vi "Convert Channels to Configuration.vi"(8 "error in":errorcluster, 10 "Conversion time":u32, 11 "Channels":T3(array[cluster]) {"RTD type" items=["User Defined"=0, "TCR3750"=2, "TCR3851"=7]}) -> (0 "error out":errorcluster, 3 "_9226 Config Data":T1 {"RTD_Type" items=["User Defined"=0, "TCR3750"=2, "TCR3851"=7]; "Degree Range" items=["Raw Ohms", "Degrees Kelvin", "Degrees Celsius", "Degrees Fahrenheit", "Degrees Rankine"]; "Conversion Time" items=["200 ms", "2.5 ms"]})   [LabVIEW 2019, in "Modules.lvlib" / "9226.lvclass"]
uses:
  9226.lvclass
  Supported RTD Types.ctl
  9226 Configuration.ctl
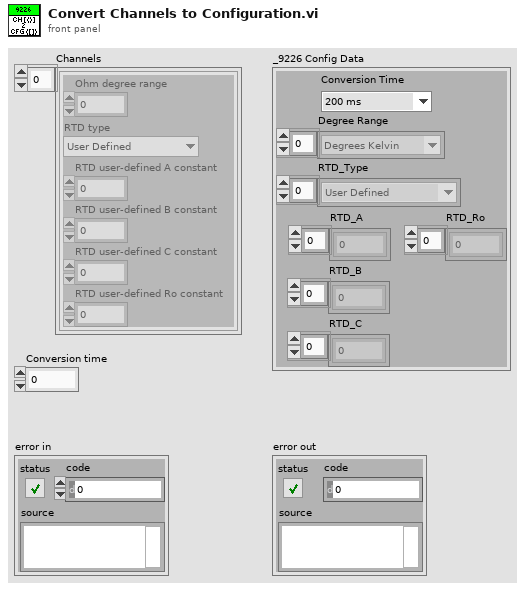
[diagram p1: front panel]
types:
  T1 = typedef "Modules.lvlib/9226.lvclass/9226 Configuration.ctl" = cluster{"Conversion Time":u16, "Degree Range":u32[], "RTD_Type":T2[], "RTD_A":dbl[], "RTD_B":dbl[], "RTD_C":dbl[], "RTD_Ro":dbl[]}
  T2 = typedef "Modules.lvlib/9226.lvclass/Supported RTD Types.ctl" = u32
  T3 = cluster{"Ohm degree range":u32, "RTD type":T2, "RTD user-defined A constant":dbl, "RTD user-defined B constant":dbl, "RTD user-defined C constant":dbl, "RTD user-defined Ro constant":dbl}[]
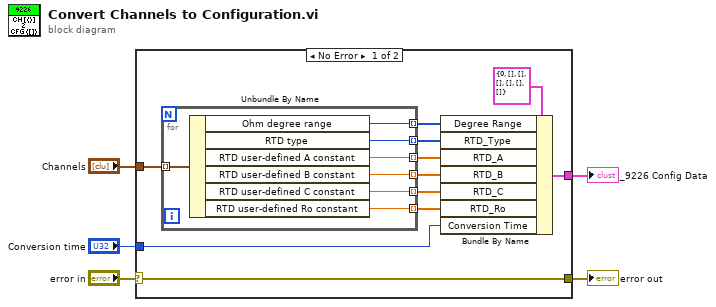
[diagram p0: block diagram]
diagram:
  n1 = case shown="No Error" "error in" {
    selector: "error in" -> [w8 w24]
    tunnel: [w8 w24] -> w3
    tunnel: "Channels" -> [w16 _]
    tunnel: "Conversion time" -> [w7 _]
    tunnel: [w9 _] -> w4
    frame No Error {
      n2 = for {
        tunnel: w16 -> [w23] mode=indexing
        tunnel: [w22] -> w15 mode=indexing
        tunnel: [w21] -> w14 mode=indexing
        tunnel: [w20] -> w13 mode=indexing
        tunnel: [w19] -> w12 mode=indexing
        tunnel: [w18] -> w11 mode=indexing
        tunnel: [w17] -> w10 mode=indexing
        n3 = Unbundle By Name(w23) -> ("Ohm degree range"=w22:u32, "RTD type"=w21:T2, "RTD user-defined A constant"=w20:dbl, "RTD user-defined B constant"=w19:dbl, "RTD user-defined C constant"=w18:dbl, "RTD user-defined Ro constant"=w17:dbl)
      }
      n4 = Bundle By Name(cluster=T1 {"Conversion Time"=0, "Degree Range"=[], "RTD_Type"=[], "RTD_A"=[], "RTD_B"=[], "RTD_C"=[], "RTD_Ro"=[]} ("_9226 Config"), "Degree Range"=w15, "RTD_Type"=w14, "RTD_A"=w13, "RTD_B"=w12, "RTD_C"=w11, "RTD_Ro"=w10, "Conversion Time"=w7) -> (w9:T1)
    }
    frame Error {
    }
  }
  "_9226 Config Data" <- w4
  "error out" <- w3
